vi "Process Mouse Data.vi"(8 "error in":errorcluster, 11 "Data":T1={"Exit"=FALSE, "States"=enum."Default", "Mouse ID"=refnum, "Mouse Data"={"axis info"={"Horizontal"=0, "Vertical"=0, "Scrolling"=0}, "Buttons"={"button 1"=FALSE, "button 2"=FALSE, "button 3"=FALSE, "button 4"=FALSE}}, "VIs"=[], "Splitters Info"=[]}) -> (0 "error out":errorcluster)   [LabVIEW 2019, in "Acquire Mouse.lvlib"]
uses:
  Acquire Mouse.lvlib
  Data.ctl
  Message Queue/State Name.ctl
  <vilib>/Utility/miscctls.llb/LVPositionTypeDef.ctl
  Status/Status.lvlib
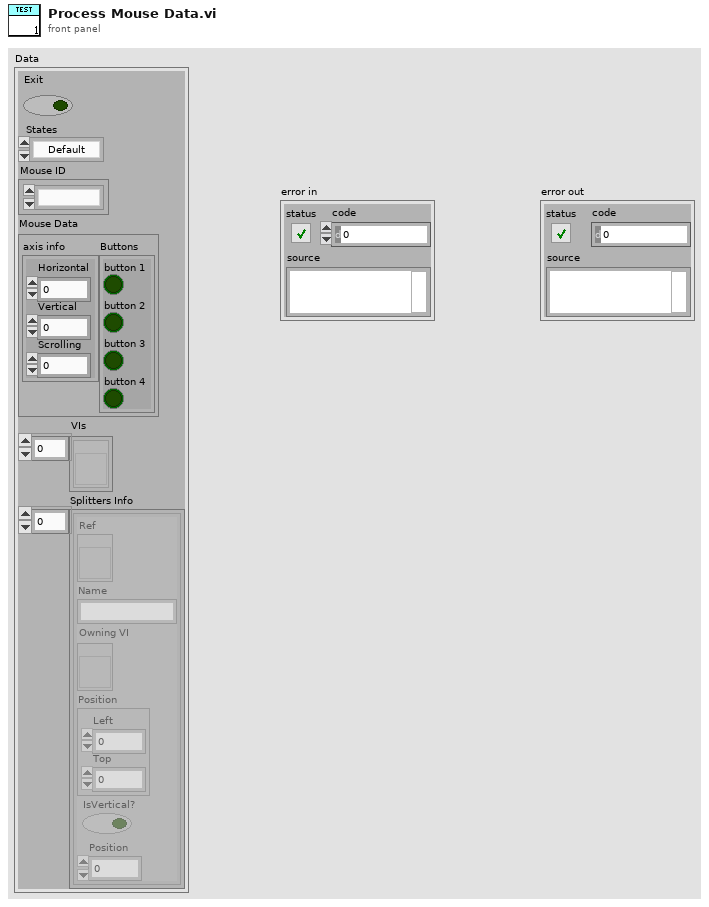
[diagram p1: front panel]
types:
  T1 = typedef "Acquire Mouse.lvlib/Data.ctl" = cluster{"Exit":bool, "States":T2, "Mouse ID":refnum<k1>, "Mouse Data":cluster{"axis info":cluster{"Horizontal":i32, "Vertical":i32, "Scrolling":i32}, "Buttons":cluster{"button 1":bool, "button 2":bool, "button 3":bool, "button 4":bool}}, "VIs":refnum<vi>[], "Splitters Info":cluster{"Ref":refnum<vi>, "Name":string, "Owning VI":refnum<vi>, "Position":T3, "IsVertical?":bool, "Position":i32}[]}
  T2 = typedef "Acquire Mouse.lvlib/State Name.ctl" = enum16{"Initialize", "Re-Initialize", "Initialize Data", "Initialize Panel", "[Event Structure] Update Data", "Add VI", "Get Splitters", "Map Splitter Pos to Coords", "Initialize Mouse", "Acquire Data", "Process Data", "Error", "Exit", "Default"}
  T3 = typedef "LVPositionTypeDef.ctl" = cluster{"Left":i32, "Top":i32}
  T4 = cluster{"Ref":refnum<vi>, "Name":string, "Owning VI":refnum<vi>, "Position":T3, "IsVertical?":bool, "Position":i32}[]
  T5 = enum32{"Bad", "Idle", "Run top level", "Running"}
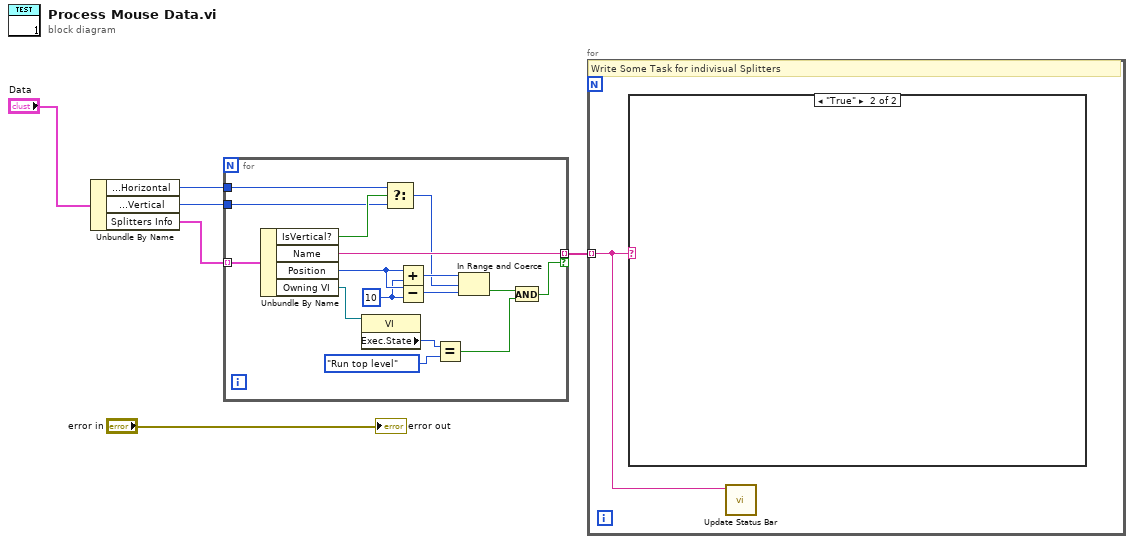
[diagram p0: block diagram]
diagram:
  n1 = Unbundle By Name("Data") -> ("Mouse Data.axis info.Horizontal"=w6:i32, "Mouse Data.axis info.Vertical"=w5:i32, "Splitters Info"=w4:T4)
  n2 = for {
    tunnel: w6 -> [w19]
    tunnel: w5 -> [w20]
    tunnel: w4 -> [w22] mode=indexing
    tunnel: [w14] -> w1 mode=indexing if=w11
    w17 = 10 ("y")
    n3 = Unbundle By Name(w22) -> ("IsVertical?"=w21:bool, "Name"=w14:string, "Position"=w18:i32, "Owning VI"=w10:refnum<vi>)
    n4 = property class="VI"(reference=w10) -> ("Exec.State"=w9:T5)  [unwired: 1 in, 2 out]
    n5 = Select(t=w19, s=w21, f=w20) -> (s? t:f=w13:i32)
    n6 = Add(x=w18, y=w17) -> (x+y=w16:i32)
    n7 = Subtract(x=w18, y=w17) -> (x-y=w15:i32)
    n8 = Equal?(x=w9, y=T5."Run top level") -> (x = y?=w7:bool)
    n9 = In Range and Coerce(upper limit=w16, x=w13, lower limit=w15) -> (In Range?=w12:bool)  [unwired: 1 out]
    n10 = And(x=w12, y=w7) -> (x .and. y?=w11:bool)
  }
  n11 = for {
    tunnel: w1 -> [w23] mode=indexing
    # "Write Some Task for indivisual Splitters"
    n12 = case shown="\"True\"" w23 {
      frame "False", Default {
      }
      frame "True" {
      }
    }
    n13 = call "Update Status Bar.vi"("Status Bar"=w23) -> ()  [unwired: 10 in, 1 out]
  }
  "error out" <- "error in"
